vi "picoquant_make_queues.vi"(8 "error in (no error)":errorcluster, 11 "picoquant_generic in":refnum<class "picoquant_generic.lvclass">) -> (0 "error out":errorcluster, 3 "picoquant_generic out":refnum<class "picoquant_generic.lvclass">)   [LabVIEW 2015, in "picoquant_generic.lvclass"]
uses:
  picoquant_generic.lvclass
  loop_notifier_tdef.ctl
  picoquant_data_tdef.ctl
  picoquant_generic.lvclass/picoquant_generic.ctl
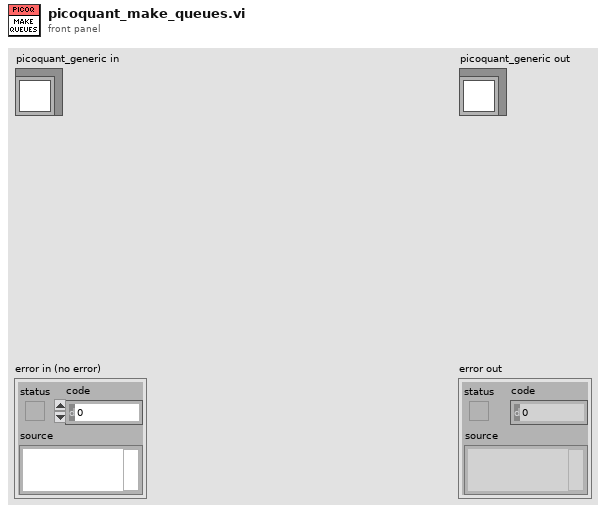
[diagram p1: front panel]
types:
  T1 = typedef "loop_notifier_tdef.ctl" = enum16{"exit"}
  T2 = typedef "picoquant_data_tdef.ctl" = cluster{"channels":u8[], "times":u64[], "sync":u64[]}
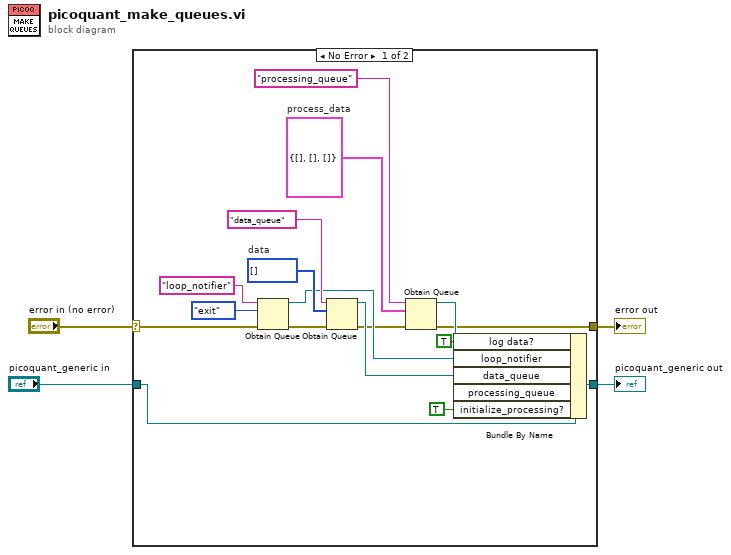
[diagram p0: block diagram]
diagram:
  n1 = case shown="No Error" "error in (no error)" {
    selector: "error in (no error)" -> [w19 w23]
    tunnel: [w7 w23] -> w3
    tunnel: [w17 w22] -> w1
    tunnel: "picoquant_generic in" -> [w18 w22]
    frame No Error {
      w9 = T2 {"channels"=[], "times"=[], "sync"=[]}  # process_data
      w14 = u32[] []  # data
      n2 = Obtain Queue(name (unnamed)="loop_notifier", element data type=loop_notifier_tdef."exit" ("loop_notifier"), error in (no error)=w19) -> (queue out=w12:refnum<queue>, error out=w16:errorcluster)  [unwired: 2 in, 1 out]
      n3 = Obtain Queue(name (unnamed)="data_queue", element data type=w14, error in (no error)=w16) -> (queue out=w13:refnum<queue>, error out=w11:errorcluster)  [unwired: 2 in, 1 out]
      n4 = Obtain Queue(name (unnamed)="processing_queue", element data type=w9, error in (no error)=w11) -> (queue out=w8:refnum<queue>, error out=w7:errorcluster)  [unwired: 2 in, 1 out]
      n5 = Bundle By Name(cluster=w18, "log data?"=TRUE, "loop_notifier"=w12, "data_queue"=w13, "processing_queue"=w8, "initialize_processing?"=TRUE) -> (w17:refnum<class "picoquant_generic.lvclass">)
    }
    frame Error {
    }
  }
  "error out" <- w3
  "picoquant_generic out" <- w1
